vi "tcp_monitor.vi"() -> ()   [LabVIEW 2022 SP3]
uses:
  <vilib>/Utility/miscctls.llb/LVPointTypeDef.ctl
  cae2d550-5c1f-4139-8f36-5e5e9cf64470.vi
  <vilib>/Utility/error.llb/Trim Whitespace One-Sided.vi
  subvis/Global 1.vi
  <vilib>/Comparison/Less/Less Functor/Less Functor.lvclass
panel:
  in  "Save":bool
  out "tcpPort":u16
  out "ip":string
  out "exit":bool
  out "area line Array":cluster{cdb[]}[](array[cluster])
  in  "Connect":bool
  in  "ping":bool
  in  "Tab Control":T1(tab)
  out "standard output":string
  out "speak_volume":cluster{"status":dbl, "volume":dbl}
  out "Frame data":string[](array[string])
  out "302 nano_heartbeat":T2
  in  "113_autoCalibration":string
  in  "100_防区":string
  in  "120_内部流地址":string
  in  "121_外部流地址":string
  in  "106_校准数据":string
  in  "110_屏蔽区":string
  in  "111_main_config":string
  in  "112_radar_area":string
  in  "set radar_area":bool
  in  "set main_config":bool
  in  "set auto calibration":bool
  in  "radar_frame_min":dbl(slide)=10.0 min=5.0 max=40.0 step=1.0 scale=5.0..40.0
  in  "joint_alarm_score":u32(slide)=150 scale=10.0..300.0
  in  "camera_alarm_score":u32(slide)=20 scale=10.0..300.0
  in  "radar_alarm_score":u32(slide)=45 scale=10.0..300.0
  in  "set声音":bool
  in  "303_volume":string="{\"code\": 303, \"data\": {\"status\": \"0\", \"speak_config\": {\"status\": 0, \"volume\": 0.6}}}"
  in  "set屏蔽区":bool
  in  "100_防区 input":string
  in  "106_校准数据 input":string
  in  "110_屏蔽区 input":string
  in  "set防区":bool
  out "DataString":string
  in  "set校准数据":bool
  in  "camera_radar_h_offset_rad":dbl(slide)=-0.01 min=-0.087 max=0.087 step=0.0001 scale=-0.087..0.087
  out "Scores":dbl[][](graph)
  out "DataTimes":dbl[][](graph)
  out "objXYs":cluster{cdb[]}[](graph)
  in  "Tab Control 2":enum32{"302", "waveforms"}(tab)=enum."waveforms"
  out "302":string
  out "200_Confidences":dbl[][](graph)
  out "301_loopTime":dbl[][](graph)
  out "heartbeat_loopTime":u32(graph)
  out "scores":string
  in  "openLogFolder":bool
  out "200":string
  out "201":string
  out "301":string
  out "path_log":path
  in  "stopButton":bool
  in  "address":string(combo)
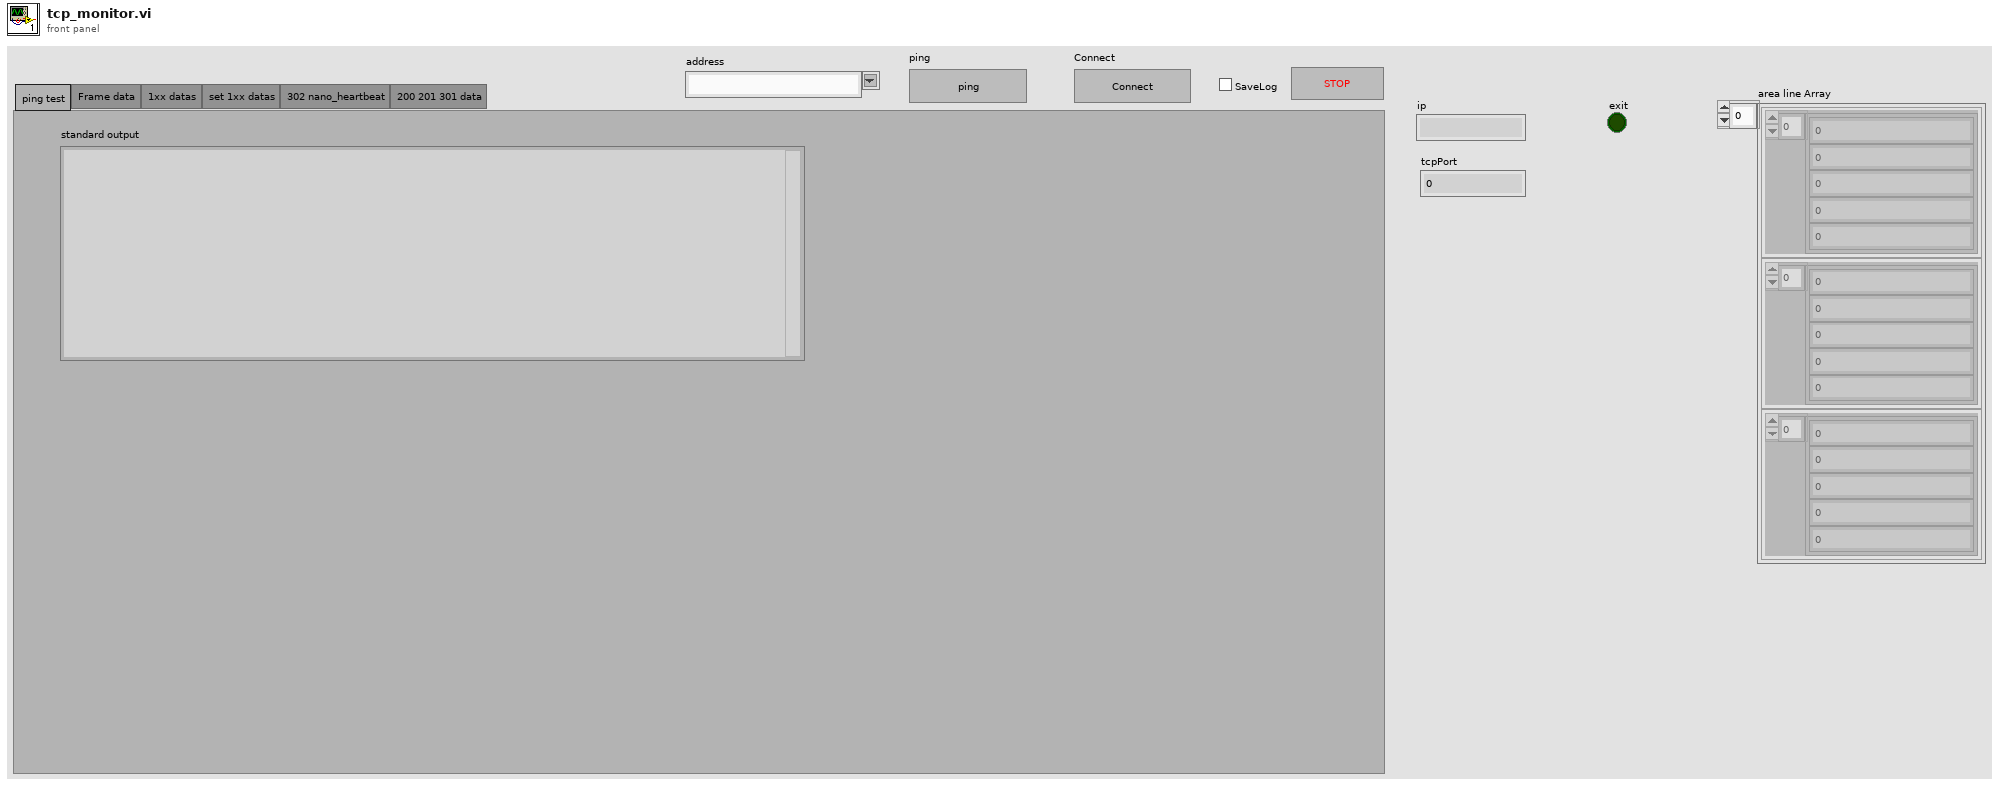
[diagram p1: front panel]
types:
  T1 = enum32{"ping test", "Frame data", "1xx datas", "set 1xx datas", "302 nano_heartbeat", "200 201 301 data"}
  T2 = cluster{"code":i32, "msg":string, "data":cluster{"reserved":cluster{"trace_score":string, "radar_latest_data_time":dbl, "camera_latest_data_time":dbl, "mcu_latest_data_time":dbl, "edition_info":cluster{"sn":string, "guard":string, "radar":string, "mcu":string}}}}
  T3 = typedef "LVPointTypeDef.ctl" = cluster{"Horizontal":i16, "Vertical":i16}
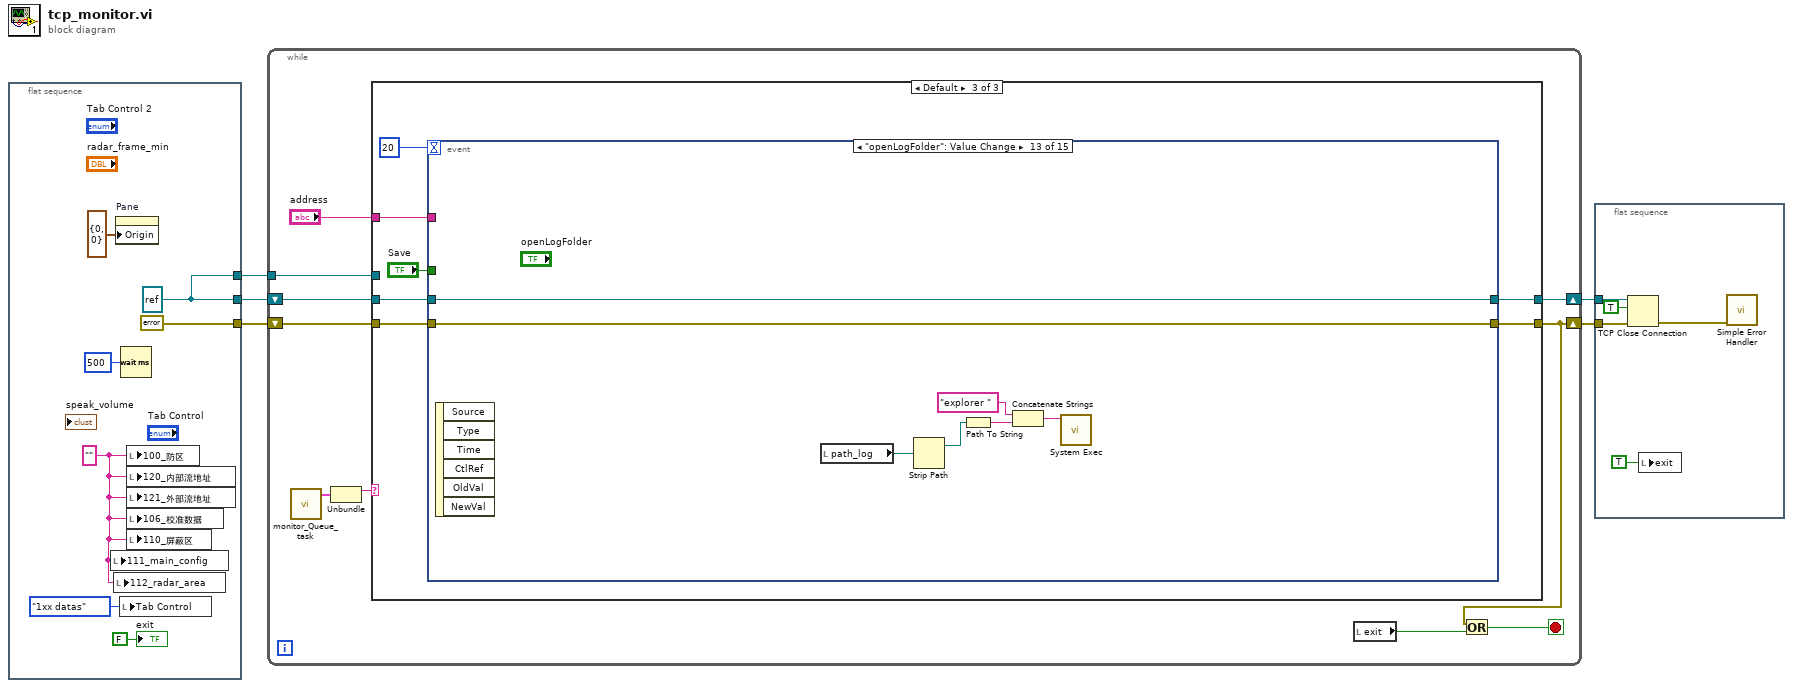
[diagram p0: block diagram]
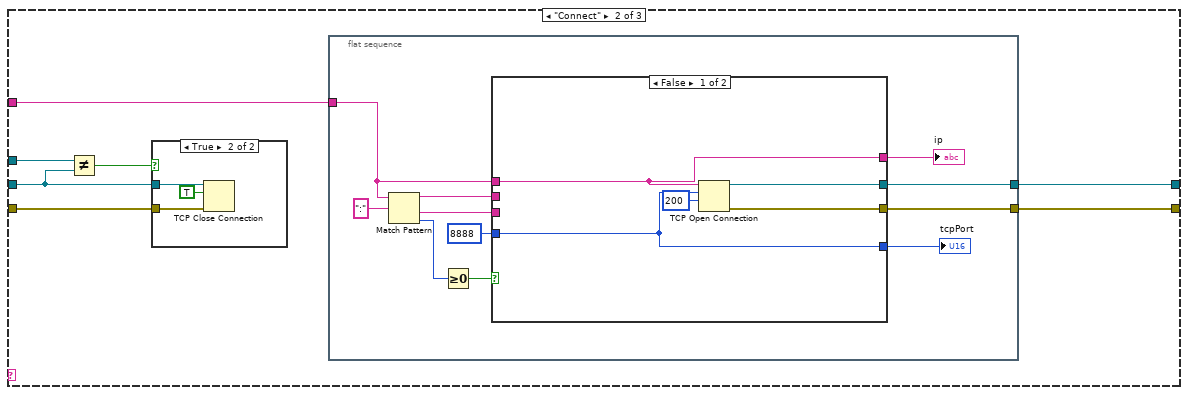
[diagram p3: hidden frame]
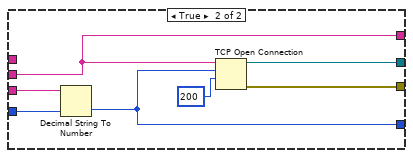
[diagram p4: hidden frame]
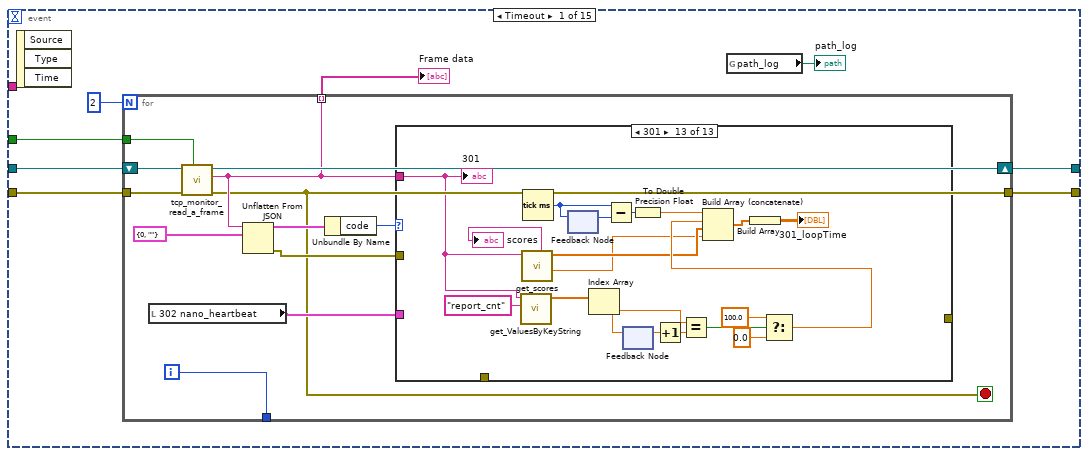
[diagram p6: hidden frame]
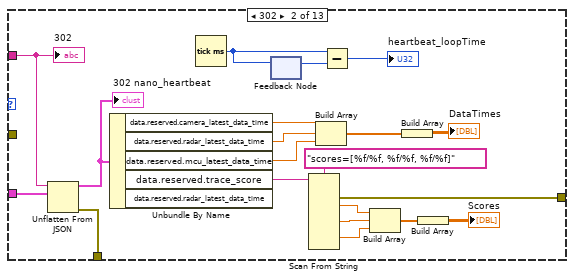
[diagram p8: hidden frame]
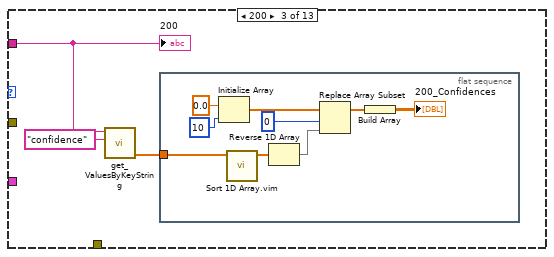
[diagram p9: hidden frame]
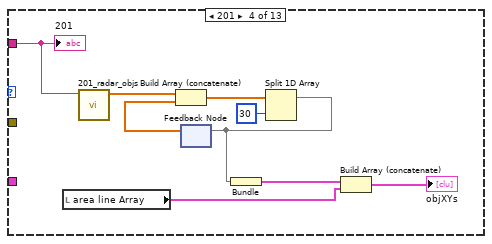
[diagram p10: hidden frame]
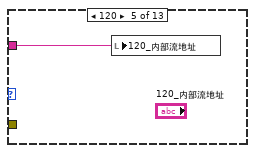
[diagram p11: hidden frame]
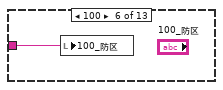
[diagram p12: hidden frame]
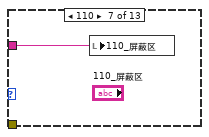
[diagram p13: hidden frame]
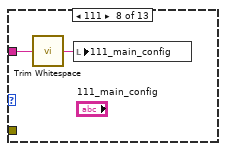
[diagram p14: hidden frame]
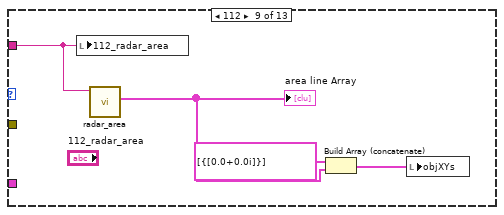
[diagram p15: hidden frame]
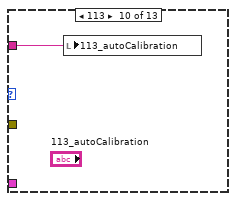
[diagram p16: hidden frame]
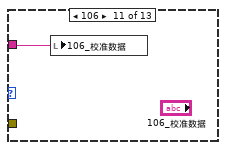
[diagram p17: hidden frame]
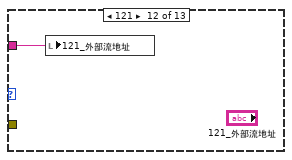
[diagram p18: hidden frame]
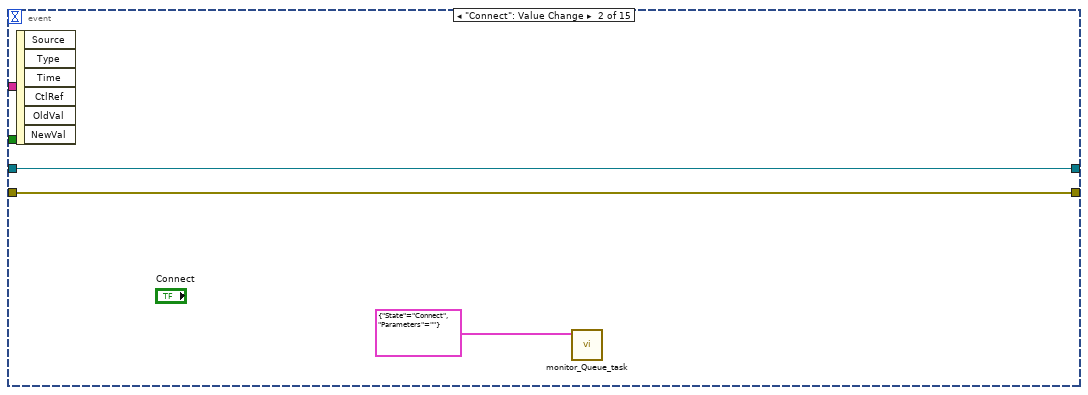
[diagram p19: hidden frame]
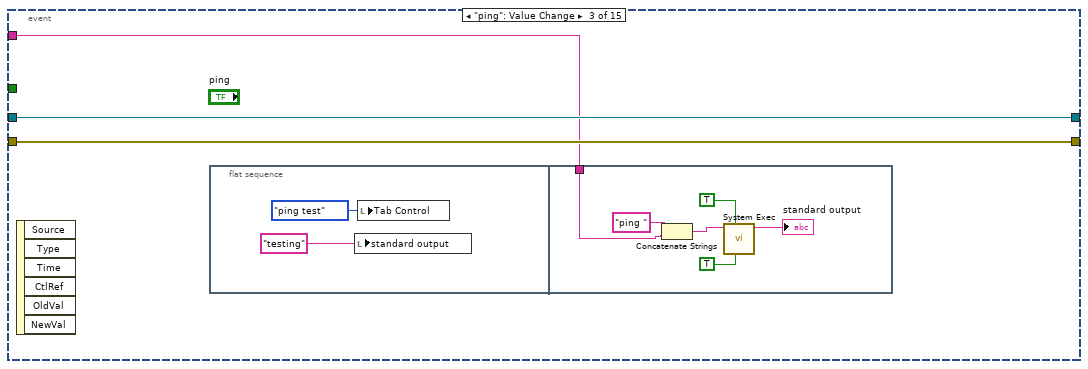
[diagram p20: hidden frame]
diagram:
  n1 = flat-sequence {
    tunnel: [w11] -> w3
    tunnel: [errorcluster {"status"=FALSE, "code"=0, "source"=""} ("error out")] -> w2
    tunnel: [w11] -> w1
    frame #0 {
      w8 = ""
      w11 = refnum<k5> refnum ("TCP Network Connection out")
      n2 = local write "111_main_config"(w8) -> ()
      n3 = local write "112_radar_area"(w8) -> ()
      n4 = property on="Pane" class="Pane"("Origin"=T3 {"Horizontal"=0, "Vertical"=0}) -> ()  [unwired: 2 in, 2 out]
      n5 = local write "Tab Control"(T1."1xx datas" ("Tab Control")) -> ()
      n6 = Wait (ms)(milliseconds to wait=u32 500) -> ()  [unwired: 1 out]
      n7 = local write "100_防区"(w8) -> ()
      n8 = local write "120_内部流地址"(w8) -> ()
      n9 = local write "121_外部流地址"(w8) -> ()
      n10 = local write "106_校准数据"(w8) -> ()
      n11 = local write "110_屏蔽区"(w8) -> ()
      "exit" <- FALSE ("stop")
    }
  }
  n12 = while {
    shift-right: [w22] -> w5
    shift-left: w3 -> [w21]
    shift-right: [w14] -> w4
    shift-left: w2 -> [w20]
    tunnel: w1 -> [w17]
    stop <- w15 stop-if-true
    n13 = call "monitor_Queue_task.vi"() -> ("taskOut"=w19:cluster{"State":string, "Parameters":string})  [unwired: 10 in, 1 out]
    n14 = Unbundle(w19) -> ("State"=w18:string)  [unwired: 1 out]
    n15 = case shown="Default" w18 {
      tunnel: [w24 w31 w64] -> w22
      tunnel: w21 -> [w24 w26 w63]
      tunnel: w20 -> [w23 w28 w62]
      tunnel: [w23 w30 w60] -> w14
      tunnel: w17 -> [_ w29 _]
      tunnel: "address" -> [_ w25 w59]
      frame "Init" {
      }
      frame "Connect" {
        n16 = Not Equal?(x=w29, y=w26) -> (x != y?=w27:bool)
        n17 = case shown="True" w27 {
          tunnel: w28 -> [_ w56]
          tunnel: w26 -> [_ w55]
          frame False {
          }
          frame True {
            n18 = TCP Close Connection(connection ID=w55, abort (F)=TRUE, error in (no error)=w56) -> ()  [unwired: 2 out]
          }
        }
        n19 = flat-sequence {
          tunnel: [w42] -> w31
          tunnel: [w41] -> w30
          tunnel: w25 -> [w38]
          frame #0 {
            n20 = Match Pattern(string=w38, regular expression=":") -> (before substring=w37:string, after substring=w36:string, offset past match=w40:i32)  [unwired: 1 in, 1 out]
            n21 = Greater Or Equal To 0?(x=w40) -> (x >= 0?=w39:bool)
            n22 = case shown="False" w39 {
              tunnel: [w47 w54] -> w42
              tunnel: [w46 w53] -> w41
              tunnel: w38 -> [w43 _]
              tunnel: w37 -> [_ w49]
              tunnel: w36 -> [_ w52]
              tunnel: u16 8888 ("remote port or service name") -> [w44 w51]
              tunnel: [w43 w49] -> w33
              tunnel: [w44 w48] -> w32
              frame False {
                n23 = TCP Open Connection(address=w43, remote port or service name=w44, timeout ms (60000)=200) -> (connection ID=w47:refnum<k5>, error out=w46:errorcluster)  [unwired: 2 in]
              }
              frame True {
                n24 = Decimal String To Number(string=w52, default (0L)=w51) -> (number=w48:u16)  [unwired: 1 in, 1 out]
                n25 = TCP Open Connection(address=w49, remote port or service name=w48, timeout ms (60000)=200) -> (connection ID=w54:refnum<k5>, error out=w53:errorcluster)  [unwired: 2 in]
              }
            }
            "ip" <- w33
            "tcpPort" <- w32
          }
        }
      }
      frame Default {
        n26 = event shown="[12] \"openLogFolder\": Value Change" {
          selector: _ -> [_ _ _ _ _ _ _ _ _ _ _ _ _ _ _]
          dyn-events: _ -> [_ _ _ _ _ _ _ _ _ _ _ _ _ _ _]
          timeout: 20 -> [_ _ _ _ _ _ _ _ _ _ _ _ _ _ _]
          tunnel: [w72 w159 w162 w175 w194 w210 w227 w240 w253 w268 w290 w306 w328 w331 w339] -> w64
          tunnel: w63 -> [w71 w159 w162 w182 w200 w212 w228 w241 w254 w271 w293 w309 w328 w331 w339]
          tunnel: w62 -> [w70 w158 w161 w176 w195 w211 w226 w239 w252 w270 w292 w308 w327 w330 w338]
          tunnel: [w67 w158 w161 w174 w193 w209 w225 w238 w251 w269 w291 w307 w327 w330 w338] -> w60
          tunnel: w59 -> [_ _ w160 _ _ _ _ _ _ _ _ _ _ _ _]
          tunnel: "Save" -> [w66 _ _ w171 w189 w207 _ _ _ w263 _ w305 _ _ _]
          event Timeout {
            n27 = event-data() -> ()  [unwired: 1 in, 3 out]
            n28 = for {
              N: 2 -> [_]
              tunnel: w70 -> [w82]
              tunnel: [w78] -> w69 mode=indexing
              shift-right: [w84] -> w72
              shift-left: w71 -> [w83]
              tunnel: [w75] -> w67
              tunnel: [w74] -> _
              tunnel: w66 -> [w73]
              i -> [w74]
              stop <- w75 stop-if-true
              n29 = local read "302 nano_heartbeat"() -> (w76:T2)
              n30 = call "tcp_monitor_read_a_frame.vi"("Save"=w73, "error in (no error)"=w82, "TCP Network Connection in"=w83) -> ("error out"=w75:errorcluster, "DataString"=w78:string, "TCP Network Connection out"=w84:refnum<k5>)  [unwired: 6 in]
              n31 = Unflatten From JSON(JSON string=w78, type and defaults=cluster{"code":i32, "msg":string} {"code"=0, "msg"=""}) -> (value=w80:cluster{"code":i32, "msg":string}, error out=w77:errorcluster)  [unwired: 5 in]
              n32 = Unbundle By Name(w80) -> ("code"=w79:i32)
              n33 = case shown="301" w79 {
                tunnel: w78 -> [_ w99 w107 w125 w126 w127 w128 w130 w134 w135 w136 w137 w141]
                tunnel: w76 -> [_ w96 _ _ _ _ _ _ _ _ _ _ _]
                tunnel: w77 -> [_ _ _ _ _ _ _ _ _ _ _ _ _]
                tunnel: [_ w94 _ _ _ _ _ _ _ _ _ _ _] -> _
                tunnel: [_ w88 _ _ _ _ _ _ _ _ _ _ _] -> _
                frame 0, Default {
                }
                frame 302 {
                  n34 = Unflatten From JSON(JSON string=w99, type and defaults=w96) -> (value=w95:T2, error out=w94:errorcluster)  [unwired: 5 in]
                  "302 nano_heartbeat" <- w95
                  n35 = Unbundle By Name(w95) -> ("data.reserved.camera_latest_data_time"=w102:dbl, "data.reserved.radar_latest_data_time"=w101:dbl, "data.reserved.mcu_latest_data_time"=w100:dbl, "data.reserved.trace_score"=w97:string)  [unwired: 1 out]
                  n36 = Tick Count (ms)() -> (millisecond timer value=w86:u32)
                  n37 = feedback-in #1(w86) -> ()
                  n38 = feedback #1() -> (w85:u32)  [unwired: 1 in]
                  n39 = Scan From String(format string="scores=[%f/%f, %f/%f, %f/%f]", input string=w97) -> (error out=w88:errorcluster, output 1=w93:dbl, output 3=w92:dbl, output 5=w91:dbl)  [unwired: 11 in, 2 out]
                  n40 = Build Array(w102, w101, w100) -> (w104:dbl[])
                  n41 = Subtract(x=w86, y=w85) -> (x-y=→"heartbeat_loopTime":u32)
                  n42 = Build Array(w93, w92, w91) -> (w90:dbl[])
                  n43 = Build Array(w104) -> (→"DataTimes":dbl[][])
                  n44 = Build Array(w90) -> (→"Scores":dbl[][])
                  "302" <- w99
                }
                frame 200 {
                  n45 = call "get_ValuesByKeyString.vi"("keyString"="confidence", "Json Input"=w107) -> ("Values"=w105:dbl[])  [unwired: 9 in]
                  n46 = flat-sequence {
                    tunnel: w105 -> [w115]
                    frame #0 {
                      n47 = Initialize Array(0.0 ("element"), 10 ("dimension size")) -> (w108:dbl[])
                      n48 = call "Sort 1D Array.vim"("unsorted array"=w115) -> ("sorted array"=w112:dbl[])  [unwired: 10 in]
                      n49 = Reverse 1D Array(array=w112) -> (reversed array=w111:dbl[])
                      n50 = Replace Array Subset(array=w108, new element=w111, index=0) -> (w113:dbl[])
                      n51 = Build Array(w113) -> (→"200_Confidences":dbl[][])
                    }
                  }
                  "200" <- w107
                }
                frame 201 {
                  n52 = local read "area line Array"() -> (w117:cluster{cdb[]}[])
                  n53 = call "201_radar_objs.vi"("201"=w125) -> ("radar_objs"=w124:cdb[])  [unwired: 10 in]
                  n54 = feedback #2() -> (w122:cdb[])  [unwired: 1 in]
                  n55 = Build Array (concatenate)(w124, w122) -> (w123:cdb[])
                  n56 = Split 1D Array(array=w123, index=30) -> (first subarray=w119:cdb[])  [unwired: 1 out]
                  n57 = feedback-in #2(w119) -> ()
                  n58 = Bundle(w119) -> (w118:cluster{cdb[]})  [unwired: 1 in]
                  n59 = Build Array (concatenate)(w118, w117) -> (→"objXYs":cluster{cdb[]}[])
                  "201" <- w125
                }
                frame 120 {
                  n60 = local write "120_内部流地址"(w126) -> ()
                }
                frame 100 {
                  n61 = local write "100_防区"(w127) -> ()
                }
                frame 110 {
                  n62 = local write "110_屏蔽区"(w128) -> ()
                }
                frame 111 {
                  n63 = call <vilib>:"Trim Whitespace.vi"("string"=w130) -> ("trimmed string"=w129:string)  [unwired: 1 in]
                  n64 = local write "111_main_config"(w129) -> ()
                }
                frame 112 {
                  n65 = local write "112_radar_area"(w134) -> ()
                  n66 = call "radar_area.vi"("String"=w134) -> ("area point Array"=w132:cluster{cdb[]}[])  [unwired: 9 in, 1 out]
                  "area line Array" <- w132
                  n67 = Build Array (concatenate)(cluster{cdb[]}[] [{[0.0+0.0i]}] ("array"), w132) -> (w133:cluster{cdb[]}[])
                  n68 = local write "objXYs"(w133) -> ()
                }
                frame 113 {
                  n69 = local write "113_autoCalibration"(w135) -> ()
                }
                frame 106 {
                  n70 = local write "106_校准数据"(w136) -> ()
                }
                frame 121 {
                  n71 = local write "121_外部流地址"(w137) -> ()
                }
                frame 301 {
                  n72 = call "get_ValuesByKeyString.vi"("keyString"="report_cnt", "Json Input"=w141) -> ("Values"=w152:dbl[])  [unwired: 9 in]
                  n73 = call "get_scores.vi"("301 Json Input"=w141) -> ("fog_coef_near"=w138:dbl, "scores"=w140:dbl[], "Json Input 2"=→"scores":string)  [unwired: 7 in, 1 out]
                  n74 = Tick Count (ms)() -> (millisecond timer value=w155:u32)
                  n75 = feedback #3() -> (w154:u32)  [unwired: 1 in]
                  n76 = feedback-in #3(w155) -> ()
                  n77 = Index Array(array=w152) -> (element=w148:dbl)  [unwired: 1 in]
                  n78 = Subtract(x=w155, y=w154) -> (x-y=w156:u32)
                  n79 = feedback-in #4(w148) -> ()
                  n80 = feedback #4() -> (w146:dbl)  [unwired: 1 in]
                  n81 = To Double Precision Float(number=w156) -> (double precision float=w150:dbl)
                  n82 = Increment(x=w146) -> (x+1=w147:dbl)
                  n83 = Equal?(x=w148, y=w147) -> (x = y?=w145:bool)
                  n84 = Select(t=100.0, s=w145, f=0.0) -> (s? t:f=w142:dbl)
                  n85 = Build Array (concatenate)(w150, w142, w140, w138) -> (w151:dbl[])
                  n86 = Build Array(w151) -> (→"301_loopTime":dbl[][])
                  "301" <- w141
                }
              }
            }
            "Frame data" <- w69
            n87 = global read "Global 1.vi" "path_log"() -> (→"path_log":path)
          }
          event "Connect": Value Change {
            n88 = event-data() -> ()  [unwired: 1 in, 6 out]
            n89 = call "monitor_Queue_task.vi"("taskInput"=cluster{"State":string, "Parameters":string} {"State"="Connect", "Parameters"=""}) -> ()  [unwired: 9 in, 2 out]
          }
          event "ping": Value Change {
            n90 = event-data() -> ()  [unwired: 1 in, 6 out]
            n91 = flat-sequence {
              tunnel: w160 -> [w165]
              frame #0 {
                n92 = local write "standard output"("testing" ("standard output")) -> ()
                n93 = local write "Tab Control"(T1."ping test" ("Tab Control")) -> ()
              }
              frame #1 {
                n94 = Concatenate Strings("ping " ("command line"), w165) -> (w166:string)
                n95 = call <vilib>:"System Exec.vi"("run minimized? (F)"=TRUE, "wait until completion? (T)"=TRUE, "command line"=w166) -> ("standard output"=→"standard output":string)  [unwired: 5 in, 3 out]
              }
            }
          }
          event "set防区": Value Change {
            n96 = event-data() -> ()  [unwired: 1 in, 6 out]
            n97 = call <vilib>:"Trim Whitespace.vi"("string"="100_防区 input") -> ("trimmed string"=w180:string)  [unwired: 1 in]
            n98 = call "tcp_monitor_gen_frame.vi"("DataString"=w180) -> ("String"=w179:string)  [unwired: 9 in, 1 out]
            n99 = TCP Write(connection ID=w182, data in=w179, 9:1000 ("timeout ms (25000)")) -> (connection ID out=w177:refnum<k5>)  [unwired: 1 in, 2 out]
            n100 = for {
              N: 1 -> [_]
              tunnel: [w184] -> w173 mode=concatenating
              shift-right: [w186] -> w175
              shift-left: w177 -> [w188]
              shift-right: [w185] -> w174
              shift-left: w176 -> [w187]
              tunnel: w171 -> [w183]
              n101 = call "tcp_monitor_read_a_frame.vi"("Save"=w183, "error in (no error)"=w187, "TCP Network Connection in"=w188) -> ("error out"=w185:errorcluster, "DataString"=w184:string, "TCP Network Connection out"=w186:refnum<k5>)  [unwired: 6 in]
            }
            "DataString" <- w173
          }
          event "set屏蔽区": Value Change {
            n102 = event-data() -> ()  [unwired: 1 in, 6 out]
            n103 = call <vilib>:"Trim Whitespace.vi"("string"="110_屏蔽区 input") -> ("trimmed string"=w199:string)  [unwired: 1 in]
            n104 = call "tcp_monitor_gen_frame.vi"("DataString"=w199) -> ("String"=w198:string)  [unwired: 9 in, 1 out]
            n105 = TCP Write(connection ID=w200, data in=w198, 9:1000 ("timeout ms (25000)")) -> (connection ID out=w196:refnum<k5>)  [unwired: 1 in, 2 out]
            n106 = for {
              N: 1 -> [_]
              tunnel: [w202] -> w190 mode=concatenating
              shift-right: [w204] -> w194
              shift-left: w196 -> [w206]
              shift-right: [w203] -> w193
              shift-left: w195 -> [w205]
              tunnel: w189 -> [w201]
              n107 = call "tcp_monitor_read_a_frame.vi"("Save"=w201, "error in (no error)"=w205, "TCP Network Connection in"=w206) -> ("error out"=w203:errorcluster, "DataString"=w202:string, "TCP Network Connection out"=w204:refnum<k5>)  [unwired: 6 in]
            }
            n108 = local write "DataString"(w190) -> ()
          }
          event "set校准数据": Value Change {
            n109 = event-data() -> ()  [unwired: 1 in, 6 out]
            n110 = flat-sequence {
              tunnel: w212 -> [w223]
              tunnel: w211 -> [w218]
              tunnel: [w217] -> w210
              tunnel: [w216] -> w209
              tunnel: "106_校准数据 input" -> [w214]
              tunnel: w207 -> [w213]
              frame #0 {
                n111 = call <vilib>:"Trim Whitespace.vi"("string"=w214) -> ("trimmed string"=w222:string)  [unwired: 1 in]
                n112 = call "tcp_monitor_gen_frame.vi"("DataString"=w222) -> ("String"=w221:string)  [unwired: 9 in, 1 out]
                n113 = TCP Write(connection ID=w223, data in=w221, 9:1000 ("timeout ms (25000)")) -> (connection ID out=w219:refnum<k5>)  [unwired: 1 in, 2 out]
                n114 = call "tcp_monitor_read_a_frame.vi"("Save"=w213, "error in (no error)"=w218, "TCP Network Connection in"=w219) -> ("error out"=w216:errorcluster, "DataString"=w215:string, "TCP Network Connection out"=w217:refnum<k5>)  [unwired: 6 in]
                n115 = local write "DataString"(w215) -> ()
              }
            }
          }
          event "set main_config": Value Change {
            n116 = event-data() -> ()  [unwired: 1 in, 6 out]
            n117 = local read "111_main_config"() -> (w224:string)
            n118 = flat-sequence {
              tunnel: [w232] -> _
              tunnel: w226 -> [w230]
              tunnel: [w231] -> w227
              tunnel: [w229] -> w225
              tunnel: w224 -> [w233]
              tunnel: w228 -> [w232]
              frame #0 {
                n119 = call <vilib>:"Trim Whitespace.vi"("string"=w233) -> ("trimmed string"=w236:string)  [unwired: 1 in]
                n120 = call "tcp_monitor_gen_frame.vi"("DataString"=w236) -> ("String"=w235:string)  [unwired: 9 in, 1 out]
                n121 = TCP Write(connection ID=w232, data in=w235, error in (no error)=w230, 9:1000 ("timeout ms (25000)")) -> (connection ID out=w231:refnum<k5>, error out=w229:errorcluster)  [unwired: 1 out]
              }
            }
          }
          event "set auto calibration": Value Change {
            (unwired) "" ("111_main_config input 2")
            n122 = event-data() -> ()  [unwired: 1 in, 6 out]
            n123 = flat-sequence {
              tunnel: [w244] -> _
              tunnel: w239 -> [w243]
              tunnel: [w246] -> w240
              tunnel: [w242] -> w238
              tunnel: "{\"code\": 113, \"msg\": \"success\", \"data\": {}}" -> [w245]
              tunnel: w241 -> [w244]
              frame #0 {
                n124 = call <vilib>:"Trim Whitespace.vi"("string"=w245) -> ("trimmed string"=w249:string)  [unwired: 1 in]
                n125 = call "tcp_monitor_gen_frame.vi"("DataString"=w249) -> ("String"=w248:string)  [unwired: 9 in, 1 out]
                n126 = TCP Write(connection ID=w244, data in=w248, error in (no error)=w243, 9:1000 ("timeout ms (25000)")) -> (connection ID out=w246:refnum<k5>, error out=w242:errorcluster)  [unwired: 1 out]
              }
            }
          }
          event "set radar_area": Value Change {
            n127 = event-data() -> ()  [unwired: 1 in, 6 out]
            n128 = local read "112_radar_area"() -> (w250:string)
            n129 = flat-sequence {
              tunnel: [w257] -> _
              tunnel: w252 -> [w256]
              tunnel: [w259] -> w253
              tunnel: [w255] -> w251
              tunnel: w250 -> [w258]
              tunnel: w254 -> [w257]
              frame #0 {
                n130 = call <vilib>:"Trim Whitespace.vi"("string"=w258) -> ("trimmed string"=w262:string)  [unwired: 1 in]
                n131 = call "tcp_monitor_gen_frame.vi"("DataString"=w262) -> ("String"=w261:string)  [unwired: 9 in, 1 out]
                n132 = TCP Write(connection ID=w257, data in=w261, error in (no error)=w256, 9:1000 ("timeout ms (25000)")) -> (connection ID out=w259:refnum<k5>, error out=w255:errorcluster)  [unwired: 1 out]
              }
            }
          }
          event "radar_alarm_score", "camera_alarm_score", "joint_alarm_score": Value Change {
            (unwired) "radar_alarm_score" ("keyString")
            n133 = event-data() -> ("CtlRef"=w267:refnum<vi>, "NewVal"=w266:u32)  [unwired: 1 in, 4 out]
            n134 = property class="Slide (strict)"(reference=w267) -> ("Label.Text"=w265:string)  [unwired: 1 in, 2 out]
            n135 = local read "111_main_config"() -> (w264:string)
            n136 = call "tcp_monitor_json_update_int.vi"("Input"=w266, "keyString"=w265, "Json Input"=w264) -> ("Json Output"=w272:string)  [unwired: 7 in, 1 out]
            n137 = disable-structure shown="Enabled" {
              disable-tunnel: w272 -> [w274 _]
              disable-tunnel: w271 -> [w278 w284]
              disable-tunnel: w270 -> [w277 w285]
              disable-tunnel: [w275 w285] -> w269
              disable-tunnel: [w276 w284] -> w268
              disable-tunnel: w263 -> [w273 _]
              frame Enabled {
                n138 = call <vilib>:"Trim Whitespace.vi"("string"=w274) -> ("trimmed string"=w283:string)  [unwired: 1 in]
                n139 = call "tcp_monitor_gen_frame.vi"("DataString"=w283) -> ("String"=w282:string)  [unwired: 9 in, 1 out]
                n140 = TCP Write(connection ID=w278, data in=w282, 9:1000 ("timeout ms (25000)")) -> (connection ID out=w280:refnum<k5>)  [unwired: 1 in, 2 out]
                n141 = call "tcp_monitor_read_a_frame.vi"("Save"=w273, "error in (no error)"=w277, "TCP Network Connection in"=w280) -> ("error out"=w275:errorcluster, "DataString"=w279:string, "TCP Network Connection out"=w276:refnum<k5>)  [unwired: 6 in]
                n142 = local write "DataString"(w279) -> ()
              }
              frame Disabled {
              }
            }
          }
          event "camera_radar_h_offset_rad": Value Change {
            n143 = event-data() -> ("CtlRef"=w289:refnum<vi>, "NewVal"=w288:dbl)  [unwired: 1 in, 4 out]
            n144 = property class="Slide (strict)"(reference=w289) -> ("Label.Text"=w287:string)  [unwired: 1 in, 2 out]
            n145 = local read "111_main_config"() -> (w286:string)
            n146 = call "tcp_monitor_json_update_double.vi"("Input"=w288, "keyString"=w287, "Json Input"=w286) -> ("Json Output"=w294:string)  [unwired: 7 in, 1 out]
            n147 = disable-structure shown="Enabled" {
              disable-tunnel: w294 -> [w297 _]
              disable-tunnel: w293 -> [w299 w303]
              disable-tunnel: w292 -> [w296 w304]
              disable-tunnel: [w295 w304] -> w291
              disable-tunnel: [w298 w303] -> w290
              frame Enabled {
                n148 = call <vilib>:"Trim Whitespace.vi"("string"=w297) -> ("trimmed string"=w302:string)  [unwired: 1 in]
                n149 = call "tcp_monitor_gen_frame.vi"("DataString"=w302) -> ("String"=w301:string)  [unwired: 9 in, 1 out]
                n150 = TCP Write(connection ID=w299, data in=w301, error in (no error)=w296, 9:1000 ("timeout ms (25000)")) -> (connection ID out=w298:refnum<k5>, error out=w295:errorcluster)  [unwired: 1 out]
              }
              frame Disabled {
              }
            }
          }
          event "set声音": Value Change {
            n151 = event-data() -> ()  [unwired: 1 in, 6 out]
            n152 = flat-sequence {
              tunnel: w309 -> [w321]
              tunnel: w308 -> [w316]
              tunnel: [w315] -> w306
              tunnel: [w314] -> w307
              tunnel: "303_volume" -> [w312]
              tunnel: w305 -> [w311]
              frame #0 {
                n153 = call <vilib>:"Trim Whitespace.vi"("string"=w312) -> ("trimmed string"=w320:string)  [unwired: 1 in]
                n154 = call "tcp_monitor_gen_frame.vi"("DataString"=w320) -> ("String"=w319:string)  [unwired: 9 in, 1 out]
                n155 = TCP Write(connection ID=w321, data in=w319, 9:1000 ("timeout ms (25000)")) -> (connection ID out=w317:refnum<k5>)  [unwired: 1 in, 2 out]
                n156 = call "tcp_monitor_read_a_frame.vi"("Save"=w311, "error in (no error)"=w316, "TCP Network Connection in"=w317) -> ("error out"=w314:errorcluster, "DataString"=w313:string, "TCP Network Connection out"=w315:refnum<k5>)  [unwired: 6 in]
                n157 = local write "DataString"(w313) -> ()
              }
            }
          }
          event "openLogFolder": Value Change {
            n158 = event-data() -> ()  [unwired: 1 in, 6 out]
            n159 = local read "path_log"() -> (w323:path)
            n160 = Strip Path(path=w323) -> (stripped path=w322:path)  [unwired: 1 out]
            n161 = Path To String(path=w322) -> (string=w326:string)
            n162 = Concatenate Strings("explorer " ("string"), w326) -> (w325:string)
            n163 = call <vilib>:"System Exec.vi"("command line"=w325) -> ()  [unwired: 7 in, 4 out]
          }
          event "stopButton": Value Change {
            n164 = event-data() -> ()  [unwired: 1 in, 6 out]
            n165 = local write "exit"(TRUE ("stop")) -> ()
          }
          event "Tab Control": Value Change {
            n166 = event-data() -> ()  [unwired: 1 in, 6 out]
            n167 = local read "106_校准数据"() -> (w335:string)
            n168 = local read "110_屏蔽区"() -> (w336:string)
            n169 = local read "100_防区"() -> (w337:string)
            n170 = call <vilib>:"Trim Whitespace.vi"("string"=w335) -> ("trimmed string"=w332:string)  [unwired: 1 in]
            n171 = call <vilib>:"Trim Whitespace.vi"("string"=w336) -> ("trimmed string"=w333:string)  [unwired: 1 in]
            n172 = call <vilib>:"Trim Whitespace.vi"("string"=w337) -> ("trimmed string"=w334:string)  [unwired: 1 in]
            n173 = local write "106_校准数据 input"(w332) -> ()
            n174 = local write "110_屏蔽区 input"(w333) -> ()
            n175 = local write "100_防区 input"(w334) -> ()
          }
        }
      }
    }
    n176 = local read "exit"() -> (w13:bool)
    n177 = Or(x=w14, y=w13) -> (x .or. y?=w15:bool)
  }
  n178 = flat-sequence {
    tunnel: w5 -> [w344]
    tunnel: w4 -> [w343]
    frame #0 {
      n179 = TCP Close Connection(connection ID=w344, abort (F)=TRUE, error in (no error)=w343) -> (error out=w342:errorcluster)  [unwired: 1 out]
      n180 = local write "exit"(TRUE ("stop")) -> ()
      n181 = call <vilib>:"Simple Error Handler.vi"("error in (no error)"=w342) -> ()  [unwired: 4 in, 5 out]
    }
  }
